vi "Get Assertion Status From Test Case.vi"(11 "Test Case Test Double in":refnum<class "Test Case Test Double.lvclass">) -> (3 "Status":T1)   [LabVIEW 2020, in "LUnit Tests.lvlib" / "Assertion Result Test.lvclass"]
uses:
  Assertion Result Test.lvclass
  source/Framework/Result Types/Assertion Result/Public/TypeDefs/Status.ctl
  Test Dummys/Test Case Test Double/Test Case Test Double.lvclass
  C:/Git/astemes-lunit/source/Framework/Test Case/LUnit Test Case.lvclass
  source/Framework/Test Case/LUnit Test Case.lvclass/LUnit Test Case.ctl
  source/Framework/Test Case/LUnit Test Case.lvclass
  source/Framework/Result Types/Case Result/Test Case Result.lvlib
  source/Framework/Result Types/Assertion Result/Assertion Result.lvlib
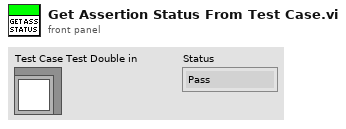
[diagram p1: front panel]
types:
  T1 = typedef "Assertion Result.lvlib/Status.ctl" = enum16{"Pass", "Fail", "Error", "Skipped", "Setup Error", "Broken", "Teardown Error"}
  T2 = typedef "Test Case Result.lvlib/Test Case Result type.ctl" = map{string, T3}
  T3 = typedef "Method Result.lvlib/Method Result type.ctl" = cluster{"Test Case":string, "Test Method Name":string, "Status":T1, "Assertion Results":T4[], "Execution time":dbl, "Result String":string}
  T4 = typedef "Assertion Result.lvlib/Assertion Result type.ctl" = cluster{"Status":T1, "Message":string, "Description":string, "Assertion Type":T5}
  T5 = typedef "Assertion Result.lvlib/Assertion Type.ctl" = enum16{"None", "Pass", "Fail", "Skip", "Pass if Equal", "Fail if Equal", "Pass if Error", "Fail if Error", "Pass if", "Fail if"}
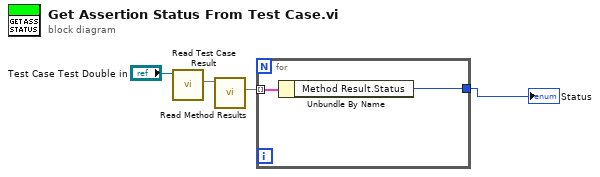
[diagram p0: block diagram]
diagram:
  n1 = call "Read Test Case Result.vi"("LUnit Test Case In"="Test Case Test Double in") -> ("Test Case Result"=w3:T2)  [unwired: 9 in, 1 out]
  n2 = call "Read Method Results.vi"("Test Case Result In"=w3) -> ("Method Results"=w4:map{string, T3})  [unwired: 9 in, 1 out]
  n3 = for {
    tunnel: [w6] -> w1
    tunnel: w4 -> [w5] mode=indexing
    n4 = Unbundle By Name(w5) -> ("Method Result.Status"=w6:T1)
  }
  "Status" <- w1
